vi "Test Case, Process File Set.vi"(8 "error in":errorcluster, 10 "index":i32) -> (0 "error out":errorcluster, 1 "Input Parameters":T1[](array[typedef]) {"Value" format="%#.3f"}, 2 "Results":T1[](array[typedef]) {"Value" format="%#.3f"}, 3 "waveform filtered":waveform(dbl)(graph)={"t0"=timestamp(3472747248.0780005 s since 1904-01-01), "dt"=2e-06, "Y"=[]})   [LabVIEW 2010]
uses:
  Generic/Waveform Attribute/Waveform Attribute Cluster.ctl
panel:
  out "File Saved":bool
  in  "Auto-increment index":bool=TRUE
  in  "Waveform Filtered Zoom":bool=TRUE
  in  "Waveform In Zoom":bool
  out "filename":path
  out "waveform":waveform(dbl)(graph)={"t0"=timestamp(3473168095.069 s since 1904-01-01), "dt"=2e-06, "Y"=[]}
  out "waveform array":waveform(dbl)={"t0"=timestamp(-9593225999.921999 s since 1904-01-01), "dt"=nan, "Y"=[]}
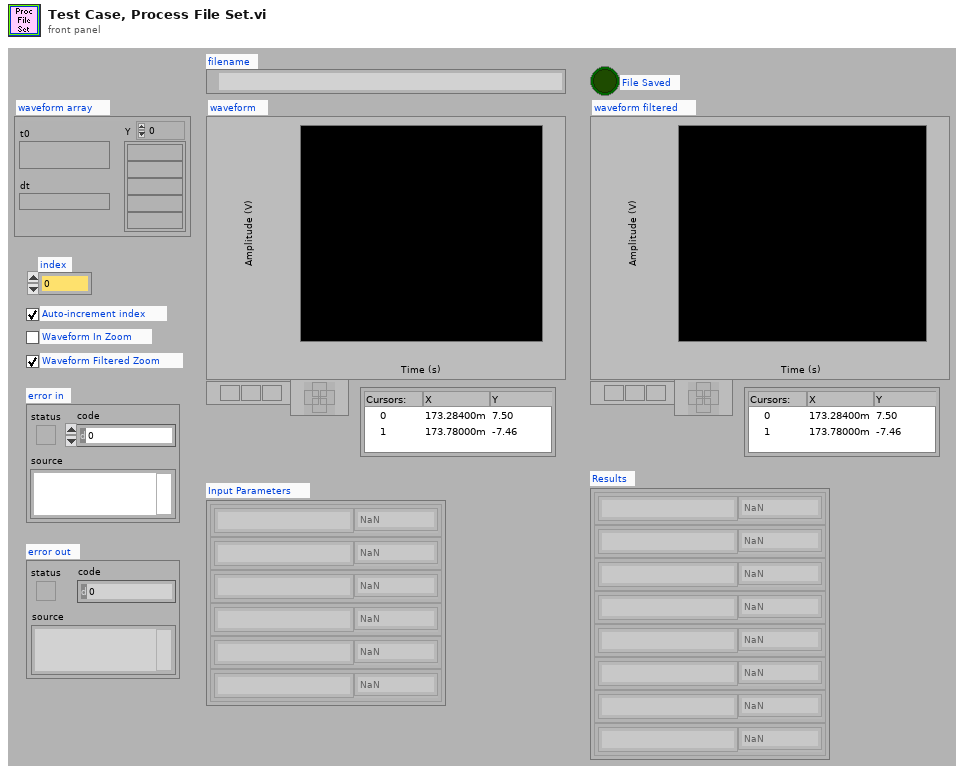
[diagram p1: front panel]
types:
  T1 = typedef "Waveform Attribute Cluster.ctl" = cluster{"Label":string, "Value":dbl}
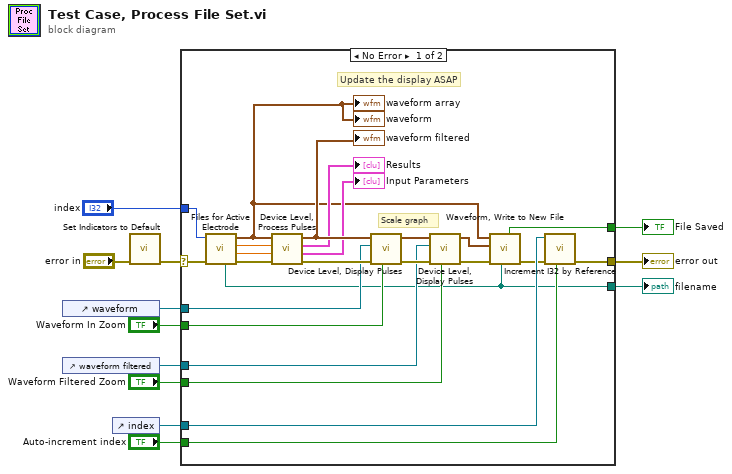
[diagram p0: block diagram]
diagram:
  n1 = control-ref of="waveform"() -> (w9:refnum<vi>)
  n2 = control-ref of="waveform filtered"() -> (w8:refnum<vi>)
  n3 = control-ref of="index"() -> (w7:refnum<vi>)
  n4 = call "Set Indicators to Default.vi"("error in"="error in") -> ("error out"=w1:errorcluster)  [unwired: 6 in]
  n5 = case shown="No Error" w1 {
    selector: w1 -> [w35 w37]
    tunnel: [w31 w37] -> w11
    tunnel: "index" -> [w32 _]
    tunnel: [w18 _] -> w10
    tunnel: w9 -> [w27 _]
    tunnel: w8 -> [w26 _]
    tunnel: w7 -> [w25 _]
    tunnel: "Waveform In Zoom" -> [w24 _]
    tunnel: "Waveform Filtered Zoom" -> [w23 _]
    tunnel: "Auto-increment index" -> [w22 _]
    tunnel: [w17 _] -> w3
    frame No Error {
      # "Scale graph"
      # "Update the display ASAP"
      n6 = call "Files for Active Electrode.vi"("error in"=w35, "index"=w32) -> ("error out"=w36:errorcluster, "Average Size"=w33:dbl, "Resistance (ohms)"=w34:dbl, "WaveformP"=w14:waveform(dbl), "Filename"=w18:path)  [unwired: 3 in]
      "waveform array" <- w14
      "waveform" <- w14
      n7 = call "Device Level, Process Pulses.vi"("error in"=w36, "Average Size"=w33, "Resistance (ohms)"=w34, "waveform"=w14) -> ("error out"=w30:errorcluster, "Input Parameters"=→"Input Parameters":T1[], "Results"=→"Results":T1[], "waveform out"=w21:waveform(dbl))  [unwired: 2 in]
      "waveform filtered" <- w21
      n8 = call "Device Level, Display Pulses.vi"("error in"=w30, "WFGraph Refnum"=w27, "waveform"=w21, "Zoom (F)"=w24) -> ("error out"=w29:errorcluster, "waveform dup"=w28:waveform(dbl))  [unwired: 5 in]
      n9 = call "Device Level, Display Pulses.vi"("error in"=w29, "WFGraph Refnum"=w26, "waveform"=w28, "Zoom (F)"=w23) -> ("error out"=w20:errorcluster, "waveform dup"=w13:waveform(dbl))  [unwired: 5 in]
      n10 = call "Waveform, Write to New File.vi"("filepath"=w18, "error in"=w20, "prc waveform"=w13, "raw waveform"=w14) -> ("error out"=w19:errorcluster, "file saved"=w17:bool)  [unwired: 2 in, 2 out]
      n11 = call "Increment I32 by Reference.vi"("error in"=w19, "dignum refnum"=w25, "enable (T)"=w22) -> ("error out"=w31:errorcluster)  [unwired: 5 in, 2 out]
    }
    frame Error {
    }
  }
  "error out" <- w11
  "filename" <- w10
  "File Saved" <- w3
